vi "Concatena_comando.vi"(2 "Opcional":string, 3 "ADRES ENETS 2":refnum<visa-resource-name>[](array[refnum]), 4 "Parametro":string, 5 "Comando":u16(ring) items=["STATUS", "GIRAR", "PARAR", "MOVER"], 6 "Dispositivo":u16(ring) items=["INDEXER", "INVERSOR", "ENCODER", "VARTRACK", "CONTROLADOR", "DOMO"], 7 "Controlador":u16(ring) items=["RA", "DEC", "CUP", "TUBO"]) -> (0 "String":string, 1 "element":refnum<visa-resource-name>)   [LabVIEW 2012]
panel:
  out "Array":bool[](array[boolean])
  out "Numeric":i32
  out "before substring":string
  # "CONTROLADOR"
  # "DISPOSITIVO"
  # "COMANDO"
  # "PARAMETRO"
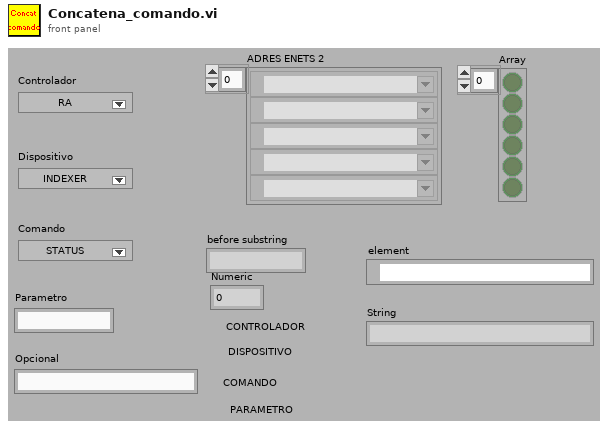
[diagram p1: front panel]
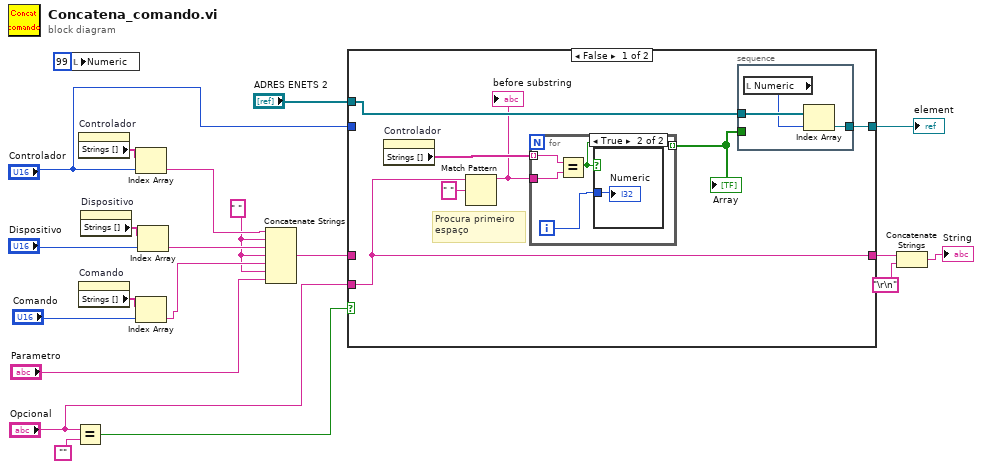
[diagram p0: block diagram]
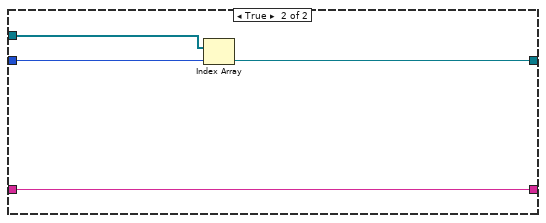
[diagram p3: hidden frame]
diagram:
  w13 = " "
  n1 = local write "Numeric"(99 ("Numeric")) -> ()
  n2 = Equal?(x="Opcional", y="") -> (x = y?=w7:bool)
  n3 = property on="Controlador" class="Ring (strict)"() -> ("Strings []"=w21:string[])  [unwired: 2 in, 2 out]
  n4 = property on="Comando" class="Ring (strict)"() -> ("Strings []"=w19:string[])  [unwired: 2 in, 2 out]
  n5 = property on="Dispositivo" class="Ring (strict)"() -> ("Strings []"=w20:string[])  [unwired: 2 in, 2 out]
  n6 = Index Array(array=w21, index="Controlador") -> (element=w14:string)
  n7 = Index Array(array=w19, index="Comando") -> (element=w15:string)
  n8 = Index Array(array=w20, index="Dispositivo") -> (element=w16:string)
  n9 = Concatenate Strings(w14, w13, w16, w13, w15, w13, "Parametro") -> (w10:string)
  n10 = case shown="False" w7 {
    tunnel: w10 -> [_ w40]
    tunnel: [w24 w40] -> w8
    tunnel: "Opcional" -> [w24 _]
    tunnel: "ADRES ENETS 2" -> [w27 w39]
    tunnel: [w28 w38] -> w3
    tunnel: "Controlador" -> [_ w37]
    frame False {
      # "Procura primeiro\nespaço"
      n11 = property on="Controlador" class="Ring (strict)"() -> ("Strings []"=w26:string[])  [unwired: 2 in, 2 out]
      n12 = Match Pattern(string=w24, regular expression=" ") -> (before substring=w25:string)  [unwired: 1 in, 3 out]
      "before substring" <- w25
      n13 = for {
        tunnel: w26 -> [w35] mode=indexing
        tunnel: w25 -> [w34]
        tunnel: [w32] -> w22 mode=indexing
        i -> [w33]
        n14 = Equal?(x=w35, y=w34) -> (x = y?=w32:bool)
        n15 = case shown="True" w32 {
          tunnel: w33 -> [_ w36]
          frame False {
          }
          frame True {
            "Numeric" <- w36
          }
        }
      }
      "Array" <- w22
      n16 = stacked-sequence {
        tunnel: [w31] -> w28
        tunnel: w27 -> [w30]
        tunnel: w22 -> [_]
        frame #0 {
          n17 = local read "Numeric"() -> (w29:i32)
          n18 = Index Array(array=w30, index=w29) -> (element=w31:refnum<visa-resource-name>)
        }
      }
    }
    frame True {
      n19 = Index Array(array=w39, index=w37) -> (element=w38:refnum<visa-resource-name>)
    }
  }
  "element" <- w3
  n20 = Concatenate Strings(w8, "\r\n") -> (→"String":string)
